vi "Position Waypoint Type Enum.vi"(8 "error in (no error)":errorcluster, 10 "String Ref":refnum<vi>, 11 "Enum Refnum":refnum<vi>) -> (0 "error out":errorcluster)   [LabVIEW 2014]
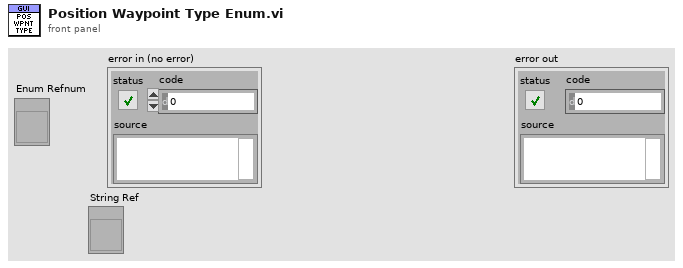
[diagram p1: front panel]
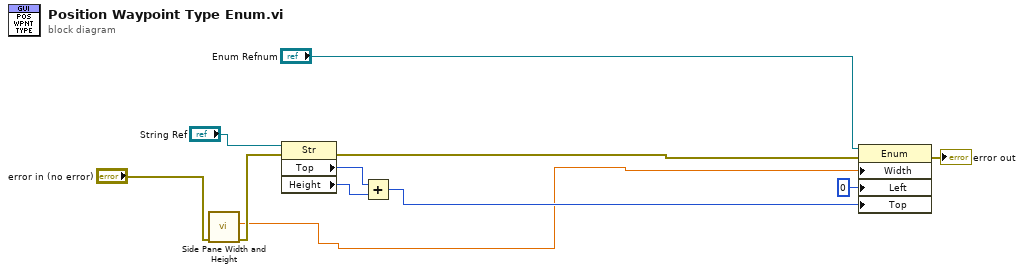
[diagram p0: block diagram]
diagram:
  n1 = call "Side Pane Width and Height.vi"("error in (no error)"="error in (no error)") -> ("error out"=w8:errorcluster, "Width"=w3:dbl)  [unwired: 8 in, 1 out]
  n2 = property class="Str"(reference="String Ref", error in=w8) -> (error out=w1:errorcluster, "Top"=w6:i32, "Height"=w5:u32)  [unwired: 1 out]
  n3 = Add(x=w6, y=w5) -> (x+y=w4:u32)
  n4 = property class="Enum"(reference="Enum Refnum", error in=w1, "Width"=w3, "Left"=0 ("Position:Left"), "Top"=w4) -> (error out=→"error out":errorcluster)  [unwired: 1 out]
